vi "ObtainRequestEvents.vi"(8 "Error":errorcluster[](array[cluster])) -> (0 "Error":errorcluster[](array[cluster]), 3 "clRequestEvents":T1)   [LabVIEW 2018, in "Visualization.lvlib" / "VisualizeBase.lvclass"]
uses:
  VisualizeBase.lvclass
  clRequestEvents.ctl
  clUserEventType.ctl
  <userlib>/NIST/NISTErrorLib/NISTErrorLib.lvlib
panel:
  # "If you want to add other Request Events, open this typedef, copy an existing event and rename it to your event name."
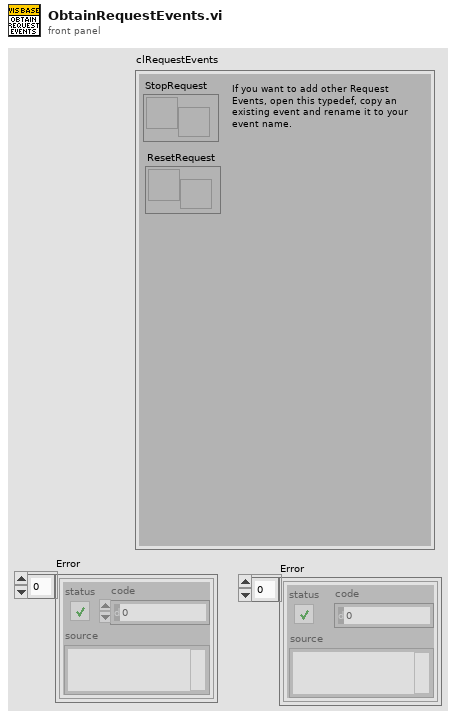
[diagram p1: front panel]
types:
  T1 = typedef "Visualization.lvlib/VisualizeBase.lvclass/clRequestEvents.ctl" = cluster{"StopRequest":refnum<user-event>, "ResetRequest":refnum<user-event>}
  T2 = typedef "Visualization.lvlib/VisualizeBase.lvclass/clUserEventType.ctl" = cluster{"BusIndex":i8, "Data":variant}
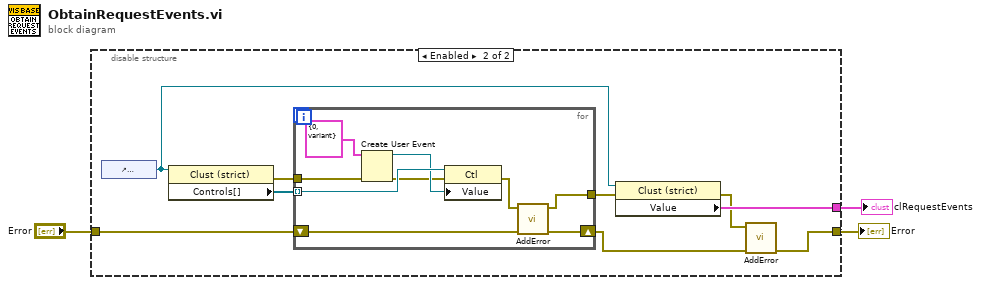
[diagram p0: block diagram]
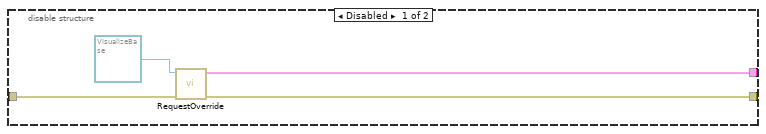
[diagram p2: hidden frame]
diagram:
  n1 = disable-structure shown="Enabled" {
    disable-tunnel: [w7 w11] -> w3
    disable-tunnel: "Error" -> [w6 w16]
    disable-tunnel: [w5 w9] -> w1
    frame Disabled {
      n2 = call-dynamic "RequestOverride.vi"("Error in"=w6, "Visualize"=refnum<class "VisualizeBase.lvclass"> refnum ("Visualization.lvlib:VisualizeBase_class.lvclass")) -> ("Error out"=w5:errorcluster[], "RequestEvents"=w7:T1)  [unwired: 8 in]
    }
    frame Enabled {
      n3 = control-ref of="clRequestEvents"() -> (w12:refnum<vi>)
      n4 = property on="Property Node" class="Clust (strict)"(reference=w12) -> (error out=w14:errorcluster, "Controls[]"=w15:refnum<vi>[])  [unwired: 1 in, 1 out]
      n5 = for {
        tunnel: w15 -> [w23] mode=indexing
        tunnel: w14 -> [w24]
        shift-right: [w18] -> w10
        shift-left: w16 -> [w19]
        tunnel: [w17] -> w13
        n6 = Create User Event(user event datatype=T2 {"BusIndex"=0, "Data"=variant} ("clEventType"), error in=w24) -> (user event=w22:refnum<user-event>, error out=w21:errorcluster)
        n7 = property class="Ctl"(reference=w23, error in=w21, "Value"=w22) -> (error out=w20:errorcluster)  [unwired: 1 out]
        n8 = call <userlib>:"AddError.vi"("ErrorArray"=w19, "error in (no error)"=w20) -> ("ErrorArray"=w18:errorcluster[], "error out"=w17:errorcluster)  [unwired: 8 in]
      }
      n9 = property on="Property Node" class="Clust (strict)"(reference=w12, error in=w13) -> (error out=w8:errorcluster, "Value"=w11:T1)  [unwired: 1 out]
      n10 = call <userlib>:"AddError.vi"("ErrorArray"=w10, "error in (no error)"=w8) -> ("ErrorArray"=w9:errorcluster[])  [unwired: 8 in, 1 out]
    }
  }
  "clRequestEvents" <- w3
  "Error" <- w1
